vi "Create or Renumber File.vi"(6 "disable buffering (F)":bool, 7 "format string (\" (%d)\")":string=" (%d)", 8 "error in (no error)":errorcluster, 11 "file path":path) -> (0 "error out":errorcluster, 3 "refnum out":refnum<file>)   [LabVIEW 2011]
doc: "Given a path to a file, this VI will create the file if it does not exist. Otherwise, this VI will create a file with the same file name but with a number appended to the end of the name. So if <b>c:\\file.txt</b> exists, then this function will create <b>c:\\file (1).txt</b>, or similar using the next available number. The directory leading to the file must alredy exist. \nIf VI returns an error then <b>actual path</b> will be the original path unmodified. Otherwise, it is the path to the newly created file.\n<b>disable buffering (F)</b> has the same meaning as on the Open\\Create\\Rename File primitive.\n<b>format string</b> must be a format string that has exactly one format code containing a %d."
panel:
  out "actual path":path
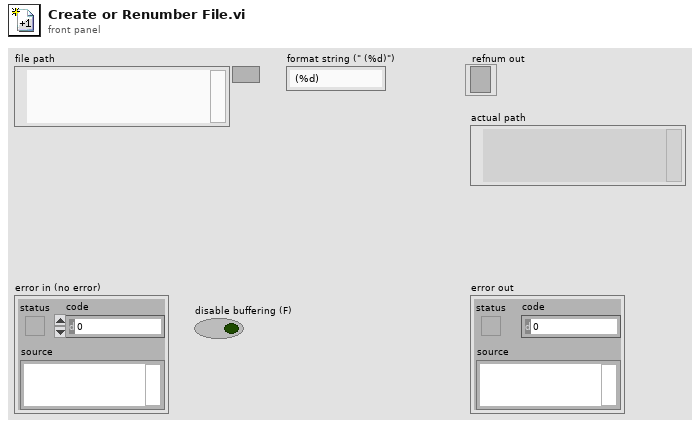
[diagram p1: front panel]
types:
  T1 = enum16{"open", "replace", "create", "open or create", "replace or create", "replace or create with confirmation"}
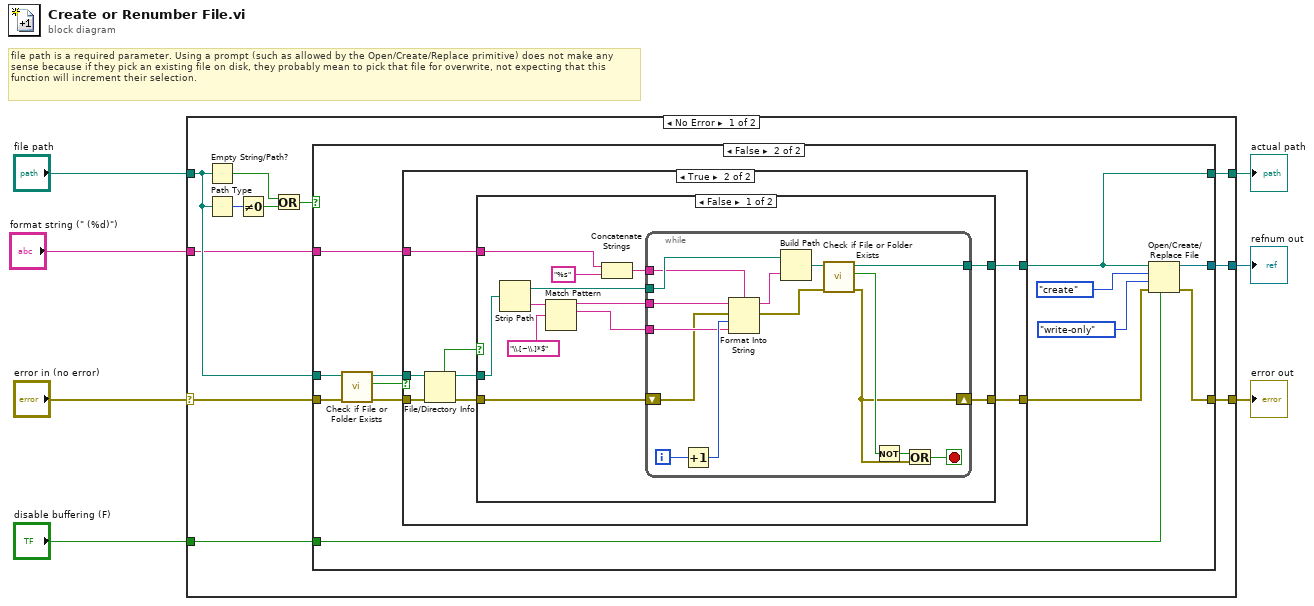
[diagram p0: block diagram]
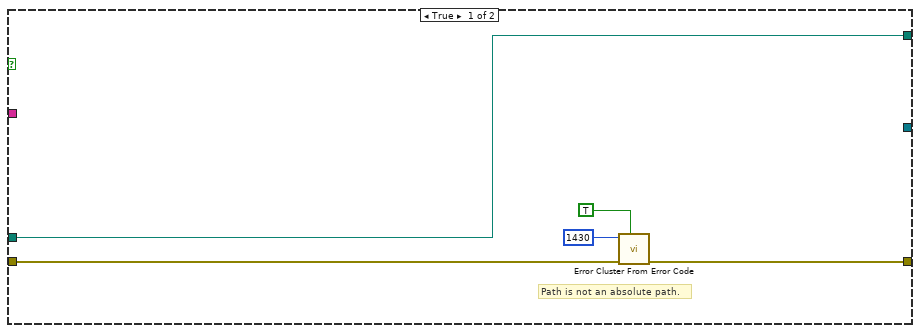
[diagram p2: hidden frame]
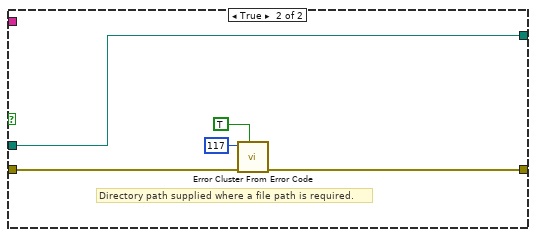
[diagram p4: hidden frame]
diagram:
  # "file path is a required parameter. Using a prompt (such as allowed by the Open/Create/Replace primitive) does not make any sense because if they pick an existing file on disk, they probably mean to pick that file for overwrite, not expecting that this function will increment their selection."
  n1 = case shown="No Error" "error in (no error)" {
    selector: "error in (no error)" -> [w15 w80]
    tunnel: "file path" -> [w10 w79]
    tunnel: "disable buffering (F)" -> [w18 _]
    tunnel: [w17 w80] -> w5
    tunnel: [w16 _] -> w4
    tunnel: [w9 w79] -> w2
    tunnel: "format string (\" (%d)\")" -> [w8 _]
    frame No Error {
      n2 = Empty String/Path?(string/path=w10) -> (empty?=w12:bool)
      n3 = Path Type(1:w10) -> (0:w14:i16)
      n4 = Not Equal To 0?(x=w14) -> (x != 0?=w13:bool)
      n5 = Or(x=w12, y=w13) -> (x .or. y?=w11:bool)
      n6 = case shown="False" w11 {
        tunnel: w18 -> [_ w36]
        tunnel: [w23 w35] -> w17
        tunnel: [_ w34] -> w16
        tunnel: w15 -> [w21 w33]
        tunnel: w10 -> [w19 w32]
        tunnel: [w19 w25] -> w9
        tunnel: w8 -> [_ w24]
        frame True {
          # "Path is not an absolute path."
          n7 = call <vilib>:"Error Cluster From Error Code.vi"("show call chain? (False)"=TRUE, "error in (no error)"=w21, "error code (0)"=1430) -> ("error out"=w23:errorcluster)  [unwired: 6 in]
        }
        frame False {
          n8 = call <vilib>:"Check if File or Folder Exists.vi"("error in (no error)"=w33, "path"=w32) -> ("error out"=w27:errorcluster, "file or folder exists?"=w29:bool, "dup path"=w28:path)  [unwired: 7 in]
          n9 = case shown="True" w29 {
            tunnel: w28 -> [w38 w46]
            tunnel: [w38 w40] -> w25
            tunnel: w27 -> [w37 w45]
            tunnel: [w37 w42] -> w26
            tunnel: w24 -> [_ w39]
            frame False {
            }
            frame True {
              n10 = File/Directory Info(path=w46, error in=w45) -> (path out=w41:path, directory=w44:bool, error out=w43:errorcluster)  [unwired: 4 out]
              n11 = case shown="False" w44 {
                tunnel: w43 -> [w58 w78]
                tunnel: [w54 w75] -> w42
                tunnel: w41 -> [w57 w74]
                tunnel: [w55 w74] -> w40
                tunnel: w39 -> [w47 _]
                frame False {
                  n12 = Strip Path(path=w57) -> (stripped path=w56:path, name=w52:string)
                  n13 = Match Pattern(string=w52, regular expression="\\.[~\\.]*$") -> (before substring=w51:string, match substring=w50:string)  [unwired: 3 out]
                  n14 = Concatenate Strings(w47, "%s" ("format string")) -> (w48:string)
                  n15 = while {
                    shift-right: [w64] -> w54
                    shift-left: w58 -> [w60]
                    tunnel: w51 -> [w73]
                    tunnel: w56 -> [w70]
                    tunnel: [w63] -> w55
                    tunnel: w50 -> [w62]
                    tunnel: w48 -> [w61]
                    i -> [w72]
                    stop <- w67 stop-if-true
                    n16 = Increment(x=w72) -> (x+1=w71:i32)
                    n17 = Format Into String(format string=w61, initial string=w73, error in=w60, w71, w62) -> (resulting string=w69:string, error out=w59:errorcluster)
                    n18 = Build Path(base path=w70, name or relative path=w69) -> (appended path=w68:path)
                    n19 = call <vilib>:"Check if File or Folder Exists.vi"("error in (no error)"=w59, "path"=w68) -> ("error out"=w64:errorcluster, "file or folder exists?"=w66:bool, "dup path"=w63:path)  [unwired: 7 in]
                    n20 = Not(x=w66) -> (.not. x?=w65:bool)
                    n21 = Or(x=w65, y=w64) -> (x .or. y?=w67:bool)
                  }
                }
                frame True {
                  # "Directory path supplied where a file path is required."
                  n22 = call <vilib>:"Error Cluster From Error Code.vi"("show call chain? (False)"=TRUE, "error in (no error)"=w78, "error code (0)"=117) -> ("error out"=w75:errorcluster)  [unwired: 6 in]
                }
              }
            }
          }
          n23 = Open/Create/Replace File(file path (use dialog)=w25, error in=w26, operation (0:open)=T1."create", access (0:read/write)=enum16{"read/write", "read-only", "write-only"}."write-only", disable buffering (F)=w36) -> (refnum out=w34:refnum<file>, error out=w35:errorcluster)  [unwired: 1 in, 1 out]
        }
      }
    }
    frame Error {
    }
  }
  "error out" <- w5
  "refnum out" <- w4
  "actual path" <- w2
